vi "Read Setpoint.vi"(10 "listen period":sgl=0.1) -> (1 "Setpoint Unit 2":string="liters/minute", 2 "Setpoint 2":sgl=1.6, 3 "Setpoint 1":sgl=80.0, 5 "Setpoint Unit 1":string="percent of flow range")   [LabVIEW 2016, in "Brooks MFC.lvclass"]
uses:
  Brooks MFC.lvclass
  Brooks MFC.lvclass/Brooks MFC.ctl
  Instance           3 21Saved   Read Setpoint .vi
panel:
  out "error out":errorcluster
  out "Brooks MFC out":refnum<class "Brooks MFC.lvclass">
  in  "Brooks MFC in":refnum<class "Brooks MFC.lvclass">
  in  "error in":errorcluster
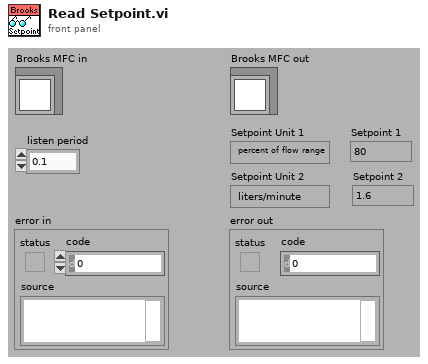
[diagram p1: front panel]
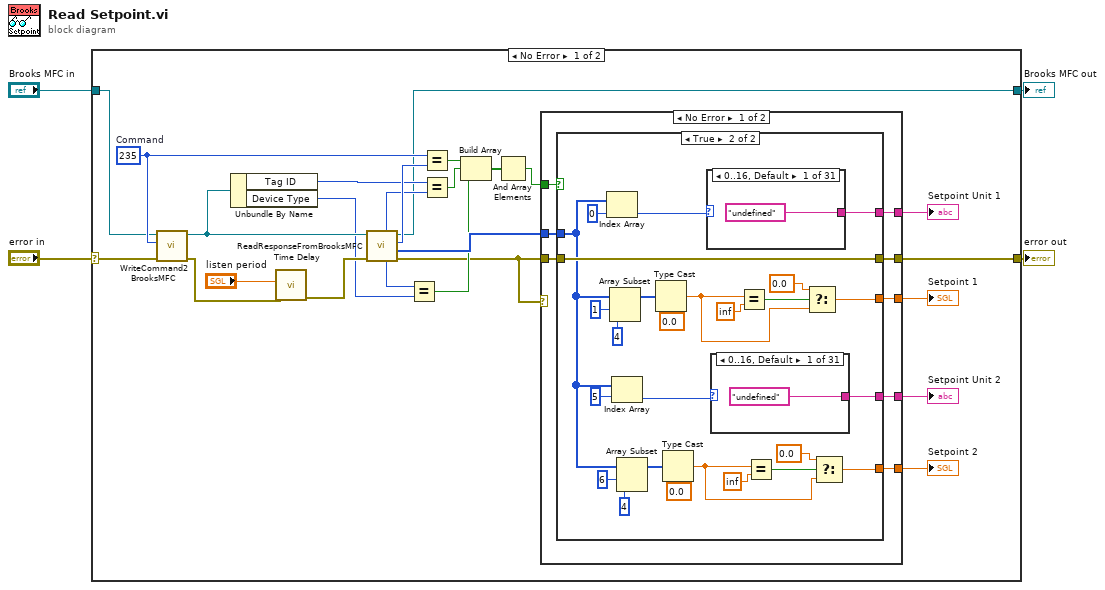
[diagram p0: block diagram]
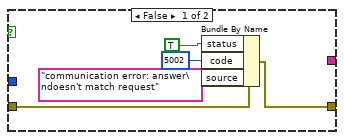
[diagram p2: hidden frame]
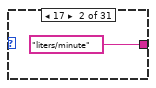
[diagram p3: hidden frame]
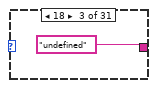
[diagram p4: hidden frame]
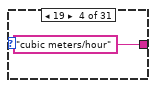
[diagram p5: hidden frame]
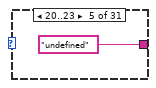
[diagram p6: hidden frame]
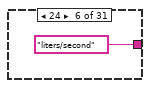
[diagram p7: hidden frame]
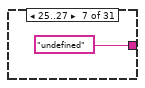
[diagram p8: hidden frame]
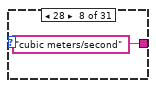
[diagram p9: hidden frame]
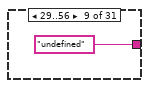
[diagram p10: hidden frame]
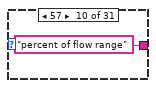
[diagram p11: hidden frame]
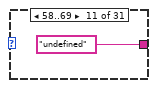
[diagram p12: hidden frame]
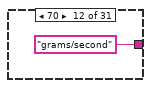
[diagram p13: hidden frame]
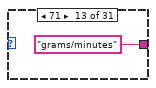
[diagram p14: hidden frame]
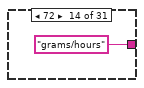
[diagram p15: hidden frame]
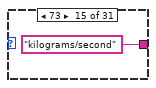
[diagram p16: hidden frame]
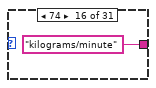
[diagram p17: hidden frame]
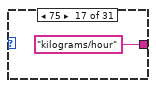
[diagram p18: hidden frame]
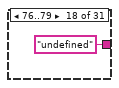
[diagram p19: hidden frame]
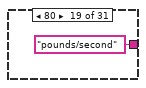
[diagram p20: hidden frame]
diagram:
  n1 = case shown="No Error" "error in" {
    selector: "error in" -> [w10 w132]
    tunnel: "Brooks MFC in" -> [w11 w133]
    tunnel: [w5 w133] -> w2
    tunnel: [w9 w132] -> w1
    frame No Error {
      w13 = u8 235  # Command
      n2 = call "WriteCommand2BrooksMFC.vi"("error in"=w10, "Command"=w13, "Brooks MFC in"=w11) -> ("error out"=w26:errorcluster, "Brooks MFC out"=w8:refnum<class "Brooks MFC.lvclass">)  [unwired: 6 in, 1 out]
      n3 = Unbundle By Name(w8) -> ("Tag ID"=w7:u32, "Device Type"=w6:u8)
      n4 = call "Time Delay"("error in (no error)"=w26, "Delay Time (s)"="listen period") -> ("error out"=w24:errorcluster)  [unwired: 9 in]
      n5 = call "ReadResponseFromBrooksMFC.vi"("error in"=w24, "Brooks MFC in"=w8) -> ("error out"=w12:errorcluster, "Data"=w29:u8[], "Command"=w27:u8, "Brooks MFC out"=w5:refnum<class "Brooks MFC.lvclass">, "device type"=w22:u8, "tag ID"=w23:u32)  [unwired: 4 in]
      n6 = Equal?(x=w22, y=w6) -> (x = y?=w19:bool)
      n7 = Equal?(x=w13, y=w27) -> (x = y?=w21:bool)
      n8 = Equal?(x=w7, y=w23) -> (x = y?=w20:bool)
      n9 = Build Array(w21, w20, w19) -> (w18:bool[])
      n10 = And Array Elements(Boolean array=w18) -> (logical AND=w17:bool)
      n11 = case shown="No Error" w12 {
        tunnel: w12 -> [w37 w131]
        tunnel: w29 -> [w36 _]
        tunnel: [w35 w131] -> w9
        tunnel: [w34 _] -> w28
        tunnel: w17 -> [w33 _]
        tunnel: [w32 _] -> w16
        tunnel: [w31 _] -> w15
        tunnel: [w30 _] -> w14
        frame No Error {
          n12 = case shown="True" w33 {
            tunnel: w36 -> [_ w47]
            tunnel: w37 -> [w40 w66]
            tunnel: [w39 w66] -> w35
            tunnel: [_ w62] -> w34
            tunnel: [_ w49] -> w32
            tunnel: [_ w45] -> w31
            tunnel: [_ w43] -> w30
            frame False {
              n13 = Bundle By Name(cluster=w40, "status"=TRUE ("Bundle Element"), "code"=5002 ("Bundle Element"), "source"="communication error: answer\ndoesn't match request") -> (w39:errorcluster)
            }
            frame True {
              n14 = Index Array(array=w47, index=0 ("Index")) -> (element=w46:u8)
              n15 = Array Subset(array=w47, index=1 ("Array Index"), length=4 ("Array Length")) -> (w61:u8[])
              n16 = Index Array(array=w47, index=5 ("Array Index")) -> (element=w44:u8)
              n17 = Array Subset(array=w47, index=6 ("Array Index"), length=4 ("Array Length")) -> (w53:u8[])
              n18 = Type Cast(type=sgl 0.0 ("x"), x=w61) -> (*(type *) &x=w59:sgl)
              n19 = Type Cast(type=sgl 0.0 ("x"), x=w53) -> (*(type *) &x=w50:sgl)
              n20 = case shown="0..16, Default" w46 {
                tunnel: ["undefined" "liters/minute" "undefined" "cubic meters/hour" "undefined" "liters/second" "undefined" "cubic meters/second" "undefined" "percent of flow range" "undefined" "grams/second" "grams/minutes" "grams/hours" "kilograms/second" "kilograms/minute" "kilograms/hour" "undefined" "pounds/second" "pounds/minute" "pounds/hour" "undefined" "cubic meters/minute" "undefined" "liters/hour" "undefined" "millimeters/second" "millimeters/minute" "millimeters/hour" "undefined" "reserved"] -> w45
                frame 0..16, Default {
                }
                frame 17 {
                }
                frame 18 {
                }
                frame 19 {
                }
                frame 20..23 {
                }
                frame 24 {
                }
                frame 25..27 {
                }
                frame 28 {
                }
                frame 29..56 {
                }
                frame 57 {
                }
                frame 58..69 {
                }
                frame 70 {
                }
                frame 71 {
                }
                frame 72 {
                }
                frame 73 {
                }
                frame 74 {
                }
                frame 75 {
                }
                frame 76..79 {
                }
                frame 80 {
                }
                frame 81 {
                }
                frame 82 {
                }
                frame 83..130 {
                }
                frame 131 {
                }
                frame 132..137 {
                }
                frame 138 {
                }
                frame 139..169 {
                }
                frame 170 {
                }
                frame 171 {
                }
                frame 172 {
                }
                frame 173..249 {
                }
                frame 250..255 {
                }
              }
              n21 = case shown="0..16, Default" w44 {
                tunnel: ["undefined" "liters/minute" "undefined" "cubic meters/hour" "undefined" "liters/second" "undefined" "cubic meters/second" "undefined" "percent of flow range" "undefined" "grams/second" "grams/minutes" "grams/hours" "kilograms/second" "kilograms/minute" "kilograms/hour" "undefined" "pounds/second" "pounds/minute" "pounds/hour" "undefined" "cubic meters/minute" "undefined" "liters/hour" "undefined" "millimeters/second" "millimeters/minute" "millimeters/hour" "undefined" "reserved"] -> w43
                frame 0..16, Default {
                }
                frame 17 {
                }
                frame 18 {
                }
                frame 19 {
                }
                frame 20..23 {
                }
                frame 24 {
                }
                frame 25..27 {
                }
                frame 28 {
                }
                frame 29..56 {
                }
                frame 57 {
                }
                frame 58..69 {
                }
                frame 70 {
                }
                frame 71 {
                }
                frame 72 {
                }
                frame 73 {
                }
                frame 74 {
                }
                frame 75 {
                }
                frame 76..79 {
                }
                frame 80 {
                }
                frame 81 {
                }
                frame 82 {
                }
                frame 83..130 {
                }
                frame 131 {
                }
                frame 132..137 {
                }
                frame 138 {
                }
                frame 139..169 {
                }
                frame 170 {
                }
                frame 171 {
                }
                frame 172 {
                }
                frame 173..249 {
                }
                frame 250..255 {
                }
              }
              n22 = Equal?(x=w59, y=sgl inf ("Single")) -> (x = y?=w64:bool)
              n23 = Equal?(x=w50, y=sgl inf ("Single")) -> (x = y?=w55:bool)
              n24 = Select(t=sgl 0.0 ("x"), s=w64, f=w59) -> (s? t:f=w62:sgl)
              n25 = Select(t=sgl 0.0 ("x"), s=w55, f=w50) -> (s? t:f=w49:sgl)
            }
          }
        }
        frame Error {
        }
      }
      "Setpoint Unit 1" <- w15
      "Setpoint Unit 2" <- w14
      "Setpoint 1" <- w28
      "Setpoint 2" <- w16
    }
    frame Error {
    }
  }
  "Brooks MFC out" <- w2
  "error out" <- w1
